vi "Format Page.vi"() -> ()   [LabVIEW 2020, in "2D Plot.lvclass"]
uses:
  <vilib>/Math Plots/2D Math Plots/2D Plot/2D Plot/2D Plot.lvclass
  <vilib>/Math Plots/2D Math Plots/2D Plot/Action String/2DMathPlot Ctrl Act Queue.ctl
  <vilib>/Math Plots/2D Math Plots/2D Plot/Action String/2DMathPlot Ctrl Act Cluster.ctl
  <vilib>/Math Plots/2D Math Plots/2D Plot/Action String/2DMathPlot State Class.ctl
  <vilib>/Math Plots/2D Math Plots/2D Plot/2D Plot/Typedef/Dialog State.ctl
  <vilib>/Math Plots/2D Math Plots/2D Plot/2D Plot/Typedef/Temp Graph State.ctl
  <vilib>/Math Plots/2D Math Plots/2D Plot/2D Plot/Typedef/Temp Graph Property Action.ctl
panel:
  in  "R Axis":string="(R-Axis)"
  in  "Axis":string[](array[string])=["(X-Axis)", "(Y-Axis)"]
  in  "Control Ref Queue":T1
  out "Format String Out":string[](array[string])
  in  "Format String In":string[](array[string])
  out "Format test string":string
  in  "Caption Texts":string[](array[string])=["Numeric Format Codes", "Absolute Time Format Codes\n(must be within %< >T)", "Relative Time Format Codes\n(must be within %< >t)"]
  in  "Item Names":string[][][](array[string])=[[["Floating point notation", "%f"], ["Scientific notation", "%e"], ["Engineering notation", "%^e"], ["Automatic notation", "%#_g"], ["SI notation", "%p"], ["Decimal", "%d"], ["Unsigned decimal", "%u"], ["Hexadecimal", "%x"], ["Octal", "%o"], ["Binary", "%b"], ["A single percent character", "%%"], ["", ""], ["", ""], ["", ""], ["", ""], ["", ""], ["", ""], ["", ""], ["", ""], ["", ""], ["", ""], ["", ""], ["", ""]], [["Absolute time container", "%< >T"], ["Abbreviated weekday name", "%a"], ["Weekday name", "%A"], ["Abbreviated month name", "%b"], ["Month name", "%B"], ["Default date and time", "%c"], ["Day of month (01-31)", "%d"], ["Hour (24-hour clock) (00-23)", "%H"], ["Hour (12-hour clock) (01-12)", "%I"], ["Day of year (001-366)", "%j"], ["Month number (01-12)", "%m"], ["Minute (00-59)", "%M"], ["AM or PM flag", "%p"], ["Seconds (00-59)", "%S"], ["Fractional seconds with <digit>\nprecision", "%<digit> u"], ["Week number (00-53) with\nSunday as the first day of week 1", "%U"], ["Weekday number (0-6)", "%w"], ["Week number (00-53) with\nMonday as the first day of week 1", "%W"], ["Locale date", "%x"], ["Locale time", "%X"], ["Year within century (00-99)", "%y"], ["Year including century", "%Y"], ["Time zone", "%Z"]], [["Relative time container", "%< >t"], ["Weeks", "%W"], ["Days", "%D"], ["Hours", "%H"], ["Minutes", "%M"], ["Seconds", "%S"], ["Fractional seconds with <digit>\nprecision", "%<digit>u"], ["A single percent character", "%%"], ["", ""], ["", ""], ["", ""], ["", ""], ["", ""], ["", ""], ["", ""], ["", ""], ["", ""], ["", ""], ["", ""], ["", ""], ["", ""], ["", ""], ["", ""]]]
  out "Advanced Tab":enum32{"Standard", "Advanced"}(tab)
  out "Time/Date Tab":enum32{"numeric", "time"}(tab) caption="Tab Control 3"
  in  "HLP_just/pad":i32(ring) items=["Pad with spaces on left", "Pad with spaces on right", "Pad with zeros on left"]
  in  "HLP_UseMinWidth":bool caption="Use minimum field width"
  in  "HLP_trailing zeros":bool caption="Hide trailing zeros"
  in  "HLP_exponent":bool caption="Exponent in multiples of 3"
  in  "Precision Type":u16(ring) items=["Digits of precision", "Significant digits"]
  in  "Digits":i32 min=0
  in  "HLP_Minimum field width":i32 caption="Minimum field width" min=0
  in  "HLP_year-new":T2(radio)
  in  "HLP_MDY 2-new":T2(radio)
  in  "HLP_HMS-new":enum32{"Radio Selection 1", "Radio Selection 2"}(radio)
  in  "HLP_Hour Type-new":enum32{"Radio Selection 1", "Radio Selection 2"}(radio)
  in  "HLP_Date Type":u16(ring)=1 caption="Date Type" items=["Custom date format", "System date format", "Date unused"]
  in  "HLP_Digits":i32 caption="Digits" min=0
  in  "HLP_Time Type":u16(ring)=1 caption="Time Type" items=["Custom time format", "System time format", "Time unused"]
  in  "Type":i32(listbox)
  in  "HLP_Revert":bool caption="Revert"
  in  "HLP_Format Code List Type":u16(ring) items=["Numeric format codes", "Relative time format codes", "Absolute time format codes"]
  out "HLP_Valid Fmt String":bool=TRUE caption="Valid"
  in  "HLP_insert format code":bool caption="Insert into Format String"
  in  "HLP_percent codes":i32(listbox) caption="Numeric Format Codes"
  in  "ODF_Format String":string caption="Format string"
  in  "HLP_AdvancedFmt2":enum32{"Default mode", "Advanced mode"}(radio)
  in  "Current Scale":u16(ring) items=["Time", "Amplitude"]
  in  "Event Registration":refnum<event-registration>
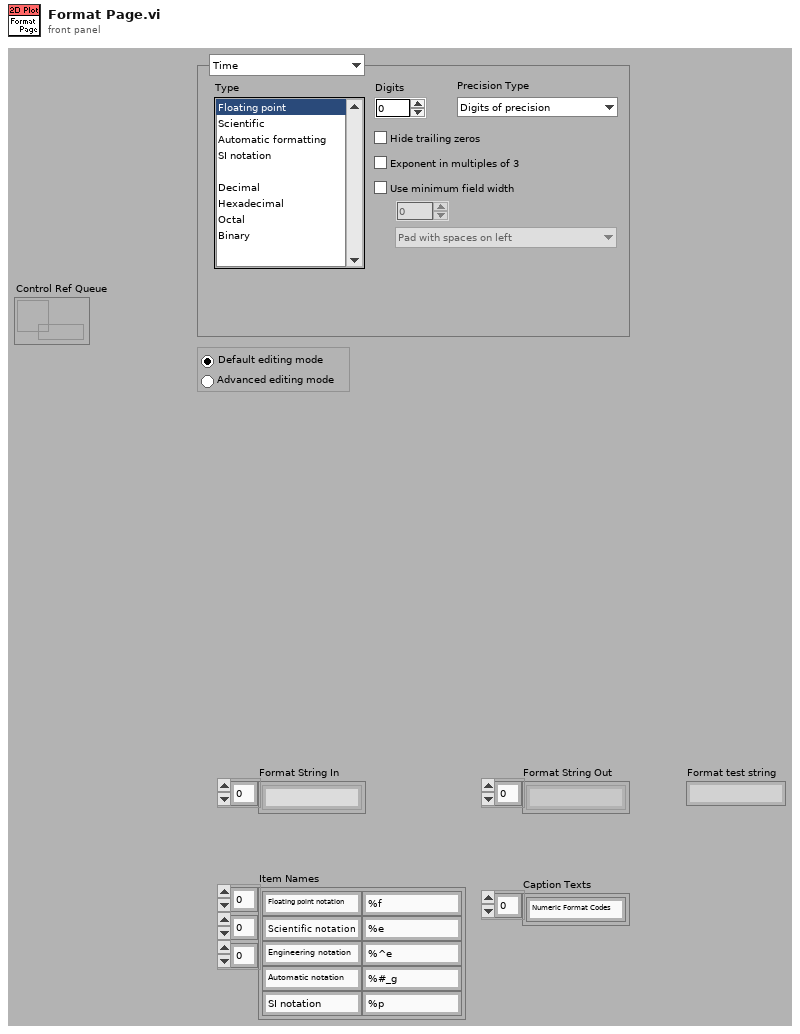
[diagram p1: front panel]
types:
  T1 = typedef "2DMathPlot Ctrl Act Queue.ctl" = refnum<queue>
  T2 = enum32{"Radio Selection 1", "Radio Selection 2", "Radio Selection 3"}
  T3 = typedef "2D Plot.lvclass/Dialog State.ctl" = enum16{"Initialize", "Read Property", "Write Property", "Idle", "Exit"}
  T4 = typedef "2D Plot.lvclass/Temp Graph State.ctl" = enum16{"Create", "Update Graph", "Update Property Only", "Get Plot Name", "Get Axis Name", "Destory"}
  T5 = typedef "2D Plot.lvclass/Temp Graph Property Action.ctl" = enum16{"Appearance Property", "Format Property", "Plots Property", "Scales Property"}
  T6 = enum16{"number", "absolute time", "relative time"}
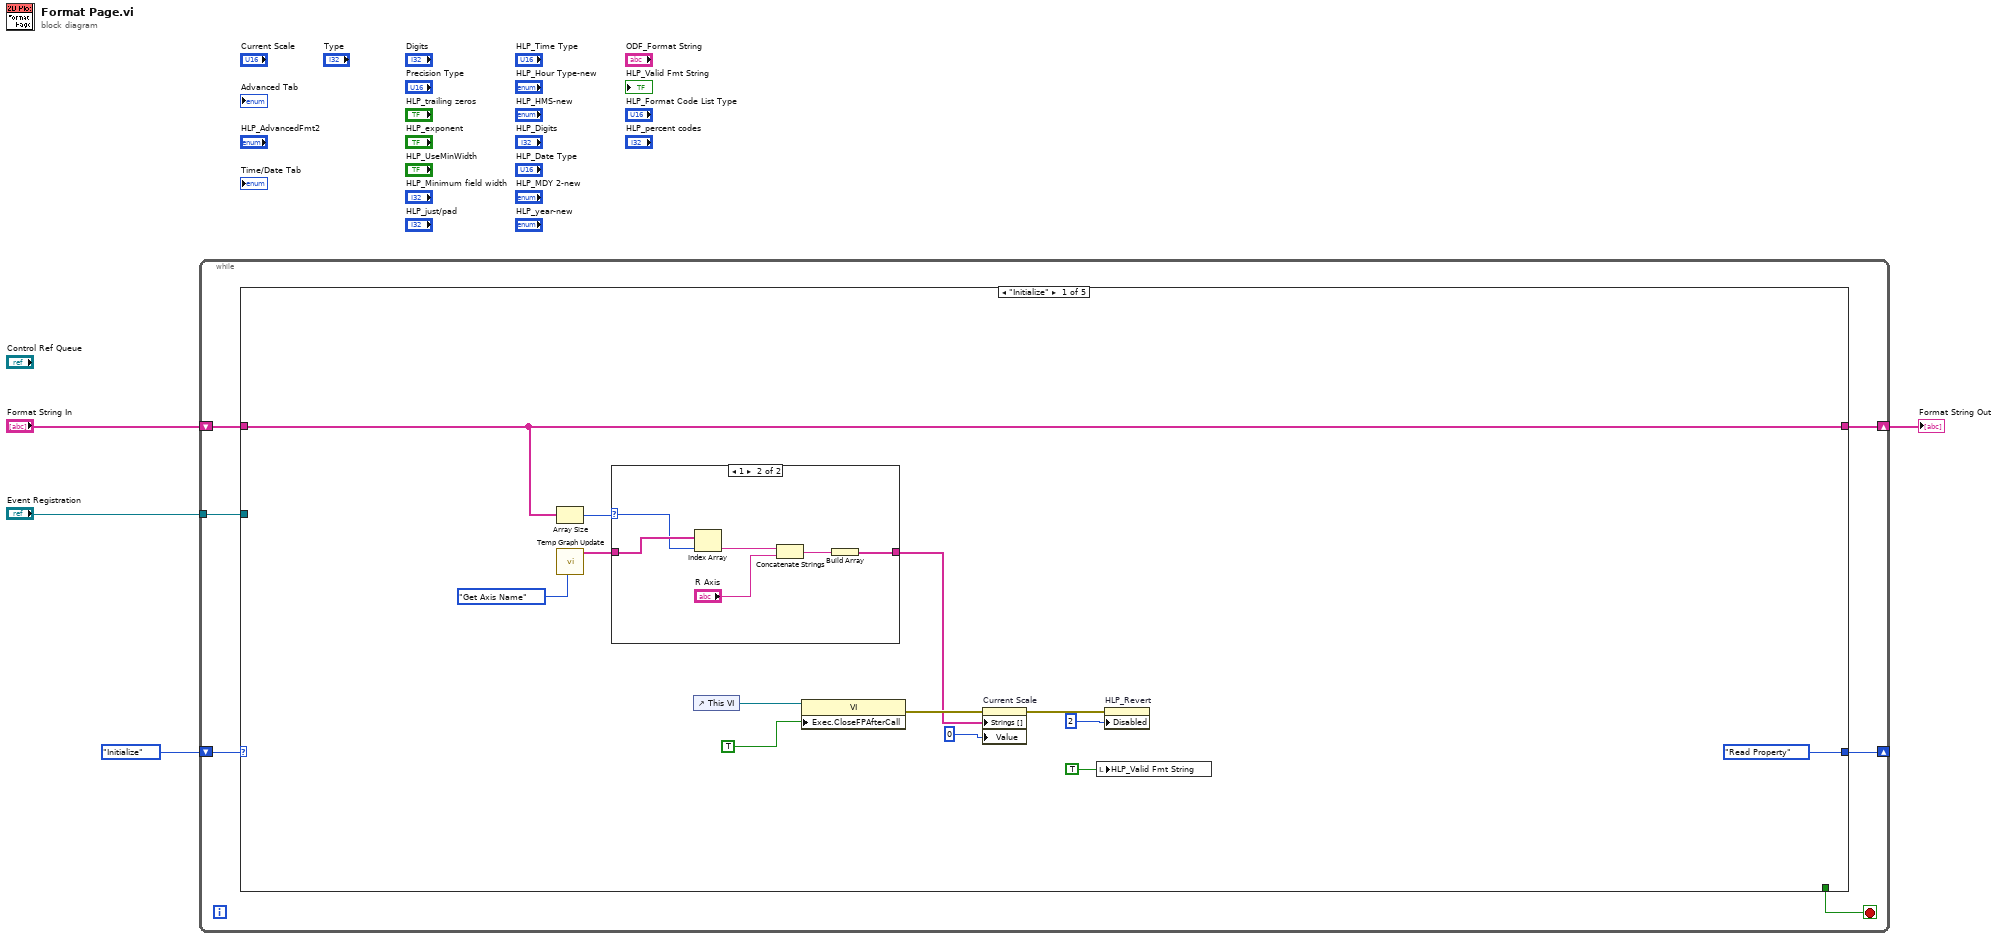
[diagram p0: block diagram]
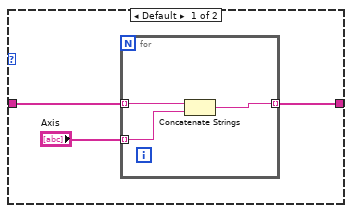
[diagram p2: hidden frame]
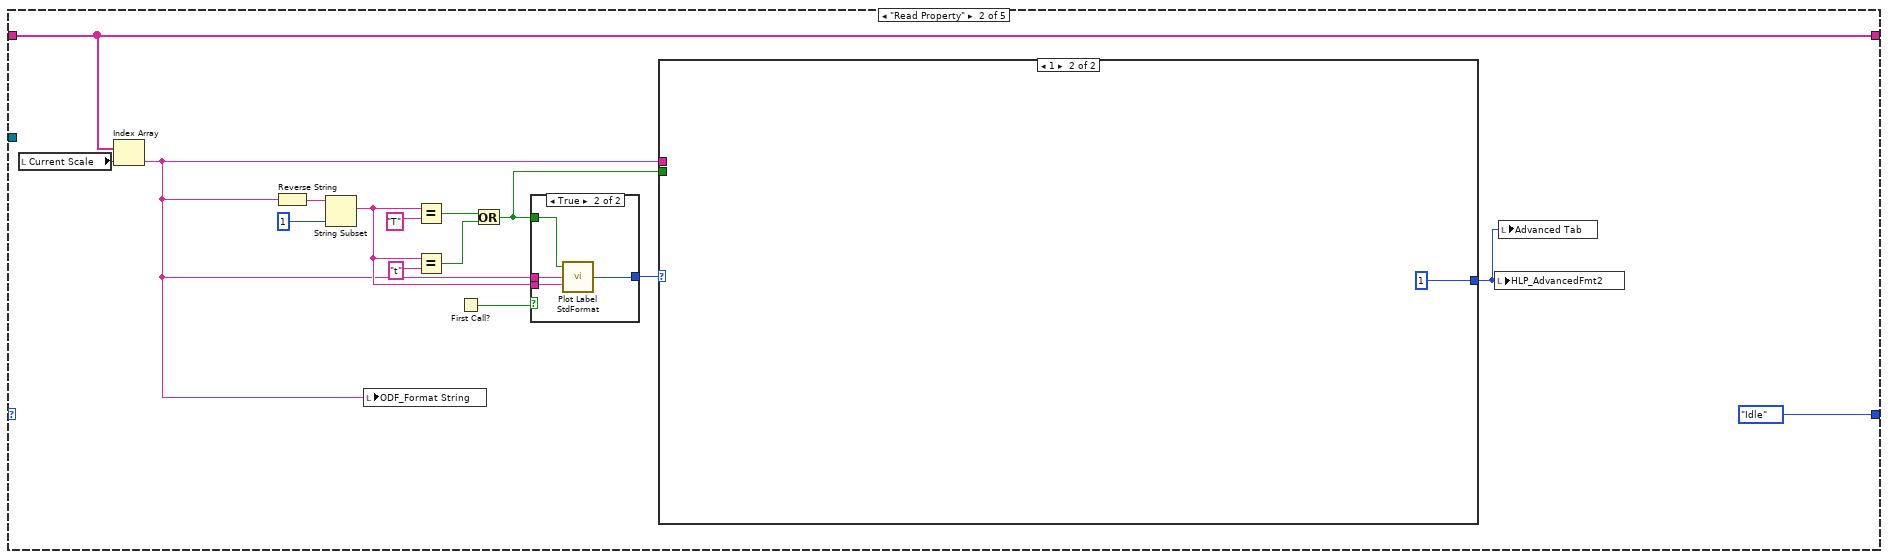
[diagram p3: hidden frame]
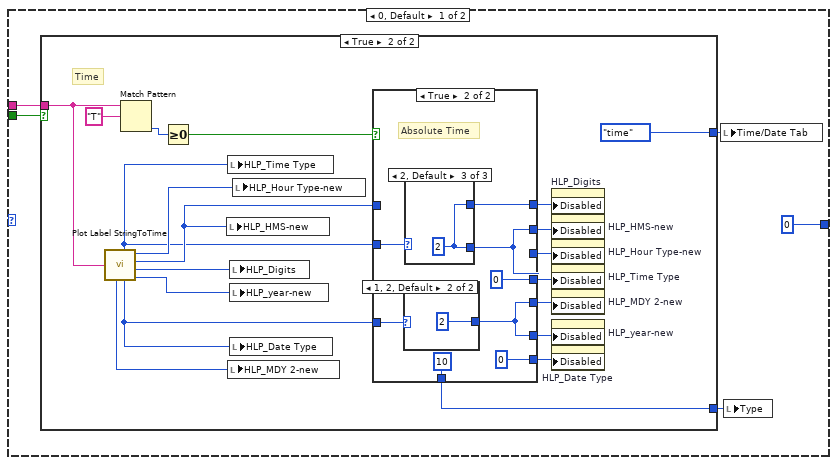
[diagram p4: hidden frame]
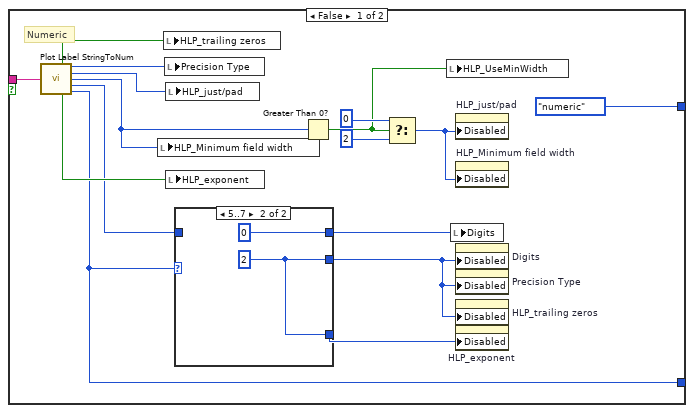
[diagram p5: hidden frame]
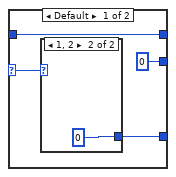
[diagram p6: hidden frame]
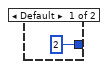
[diagram p7: hidden frame]
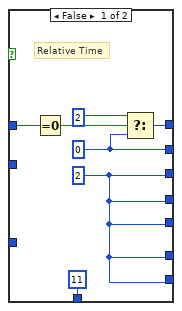
[diagram p8: hidden frame]
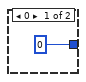
[diagram p9: hidden frame]
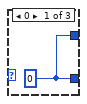
[diagram p10: hidden frame]
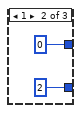
[diagram p11: hidden frame]
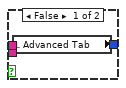
[diagram p12: hidden frame]
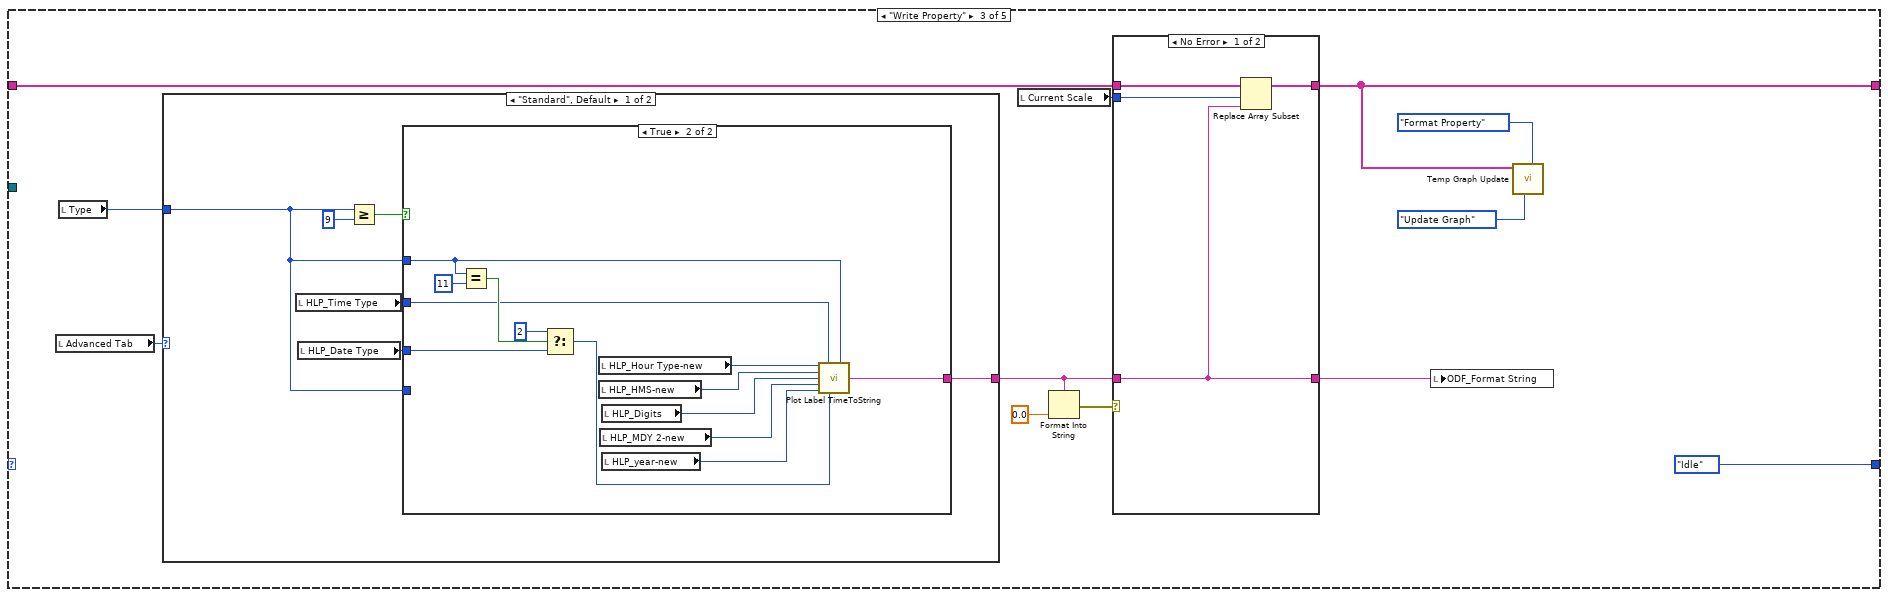
[diagram p13: hidden frame]
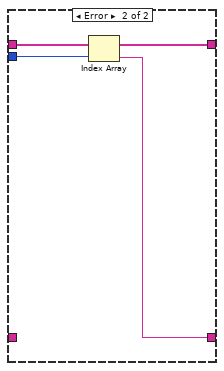
[diagram p14: hidden frame]
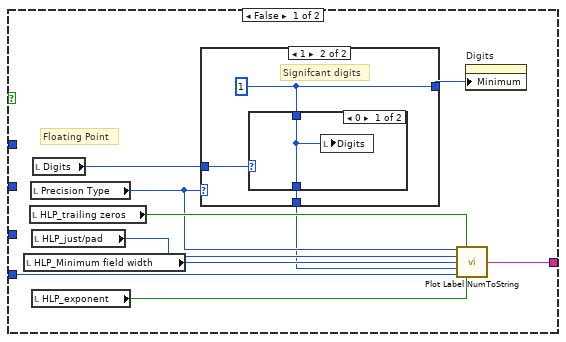
[diagram p15: hidden frame]
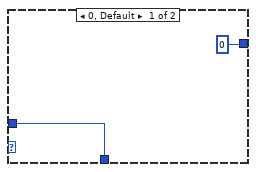
[diagram p16: hidden frame]
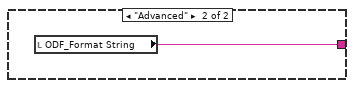
[diagram p18: hidden frame]
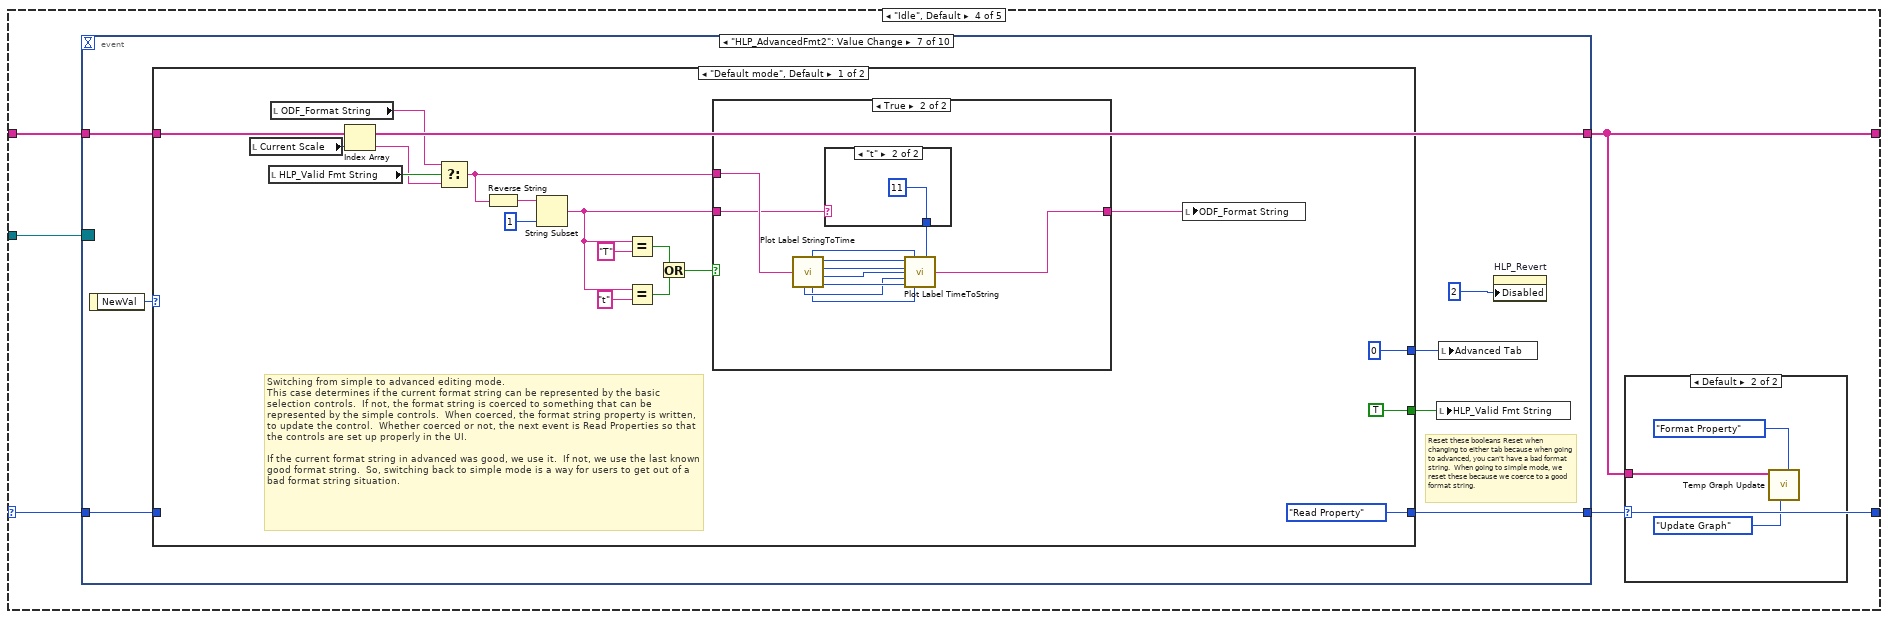
[diagram p19: hidden frame]
diagram:
  n1 = while {
    shift-right: [w5] -> w2
    shift-left: "Format String In" -> [w10]
    shift-right: [w6] -> _
    shift-left: Dialog_State."Initialize" ("Enum") -> [w7]
    tunnel: "Event Registration" -> [w8]
    stop <- w9 stop-if-true
    n2 = case shown="\"Initialize\"" w7 {
      selector: w7 -> [_ _ _ w185 _]
      tunnel: w10 -> [w15 w49 w130 w187 w410]
      tunnel: [w15 w49 w127 w184 w410] -> w5
      tunnel: [Dialog_State."Read Property" ("Enum") Dialog_State."Idle" ("Enum") Dialog_State."Idle" ("Enum") w183 Dialog_State."Exit" ("Enum")] -> w6
      tunnel: [_ _ _ _ TRUE] -> w9
      tunnel: w8 -> [_ _ _ w186 _]
      frame "Initialize" {
        n3 = Array Size(array=w15) -> (size(s)=w12:i32)
        n4 = call <vilib>:"Temp Graph Update.vi"("State"=Temp_Graph_State."Get Axis Name") -> ("Item Strings"=w14:string[])  [unwired: 4 in, 6 out]
        n5 = case shown="1" w12 {
          selector: w12 -> [_ w34]
          tunnel: w14 -> [w26 w35]
          tunnel: [w24 w30] -> w13
          frame Default {
            n6 = for {
              tunnel: w26 -> [w29] mode=indexing
              tunnel: "Axis" -> [w28] mode=indexing
              tunnel: [w27] -> w24 mode=indexing
              n7 = Concatenate Strings(w29, w28) -> (w27:string)
            }
          }
          frame 1 {
            n8 = Index Array(array=w35, index=w34) -> (element=w33:string)
            n9 = Concatenate Strings(w33, "R Axis") -> (w31:string)
            n10 = Build Array(w31) -> (w30:string[])
          }
        }
        n11 = control-ref of="This VI"() -> (w23:refnum<vi>)
        n12 = property class="VI"(reference=w23, "Exec.CloseFPAfterCall"=TRUE ("Execution:Close After Call")) -> (error out=w18:errorcluster)  [unwired: 1 in, 1 out]
        n13 = property on="Current Scale" class="Ring (strict)"(error in=w18, "Strings []"=w13, "Value"=u16 0) -> (error out=w17:errorcluster)  [unwired: 1 in, 1 out]
        n14 = local write "HLP_Valid Fmt String"(TRUE ("HLP_Valid Fmt String")) -> ()
        n15 = property on="HLP_Revert" class="Bool"(error in=w17, "Disabled"=u8 2) -> ()  [unwired: 1 in, 2 out]
      }
      frame "Read Property" {
        n16 = local read "Current Scale"() -> (w50:u16)
        n17 = Index Array(array=w49, index=w50) -> (element=w39:string)
        n18 = Reverse String(1:w39) -> (0:w44:string)
        n19 = String Subset(string=w44, length (rest)=1 ("length (rest)")) -> (substring=w48:string)  [unwired: 1 out]
        n20 = local write "ODF_Format String"(w39) -> ()
        n21 = Equal?(x=w48, y="T") -> (x = y?=w46:bool)
        n22 = Equal?(x=w48, y="t") -> (x = y?=w47:bool)
        n23 = First Call?() -> (First Call?: T/F=w41:bool)
        n24 = Or(x=w46, y=w47) -> (x .or. y?=w38:bool)
        n25 = case shown="True" w41 {
          tunnel: w48 -> [_ w124]
          tunnel: w38 -> [_ w126]
          tunnel: w39 -> [_ w125]
          tunnel: [w122 w123] -> w40
          frame False {
            n26 = local read "Advanced Tab"() -> (w122:enum32{"Standard", "Advanced"})
          }
          frame True {
            n27 = call <vilib>:"Plot Label StdFormat.vi"("Time Type"=w124, "Format String"=w125, "Type (false = numeric)"=w126) -> ("Custom"=w123:i32)
          }
        }
        n28 = case shown="1" w40 {
          tunnel: w39 -> [w55 _]
          tunnel: w38 -> [w54 _]
          tunnel: [0 1] -> w37
          frame 0, Default {
            n29 = case shown="True" w54 {
              tunnel: w55 -> [w71 w97]
              tunnel: [w64 w88] -> w53
              tunnel: [enum32{"numeric", "time"}."numeric" ("Time/Date Tab") enum32{"numeric", "time"}."time" ("Time/Date Tab")] -> w52
              frame False {
                # "Numeric"
                n30 = call <vilib>:"Plot Label StringToNum.vi"("Format String"=w71) -> ("Hide trailing zeros"=w70:bool, "Digit Type"=w68:i32, "just/pad"=w67:i32, "Minimum Field Width"=w59:i32, "Digits of Precision"=w66:i32, "exponent"=w69:bool, "Numeric Format"=w64:i32)  [unwired: 8 out]
                n31 = local write "HLP_Minimum field width"(w59) -> ()
                n32 = local write "HLP_trailing zeros"(w70) -> ()
                n33 = local write "Precision Type"(w68) -> ()
                n34 = local write "HLP_just/pad"(w67) -> ()
                n35 = local write "HLP_exponent"(w69) -> ()
                n36 = case shown="5..7" w64 {
                  selector: w64 -> [w73 _]
                  tunnel: [u8 0 w78] -> w63
                  tunnel: w66 -> [w74 _]
                  tunnel: [w74 0 ("Digits of Precision")] -> w65
                  tunnel: [w72 w78] -> w62
                  frame Default {
                    n37 = case shown="1, 2" w73 {
                      tunnel: [u8 2 u8 0] -> w72
                      frame Default {
                      }
                      frame 1, 2 {
                      }
                    }
                  }
                  frame 5..7 {
                    w78 = u8 2
                  }
                }
                n38 = Greater Than 0?(x=w59) -> (x > 0?=w58:bool)
                n39 = Select(t=u8 0, s=w58, f=u8 2) -> (s? t:f=w57:u8)
                n40 = local write "HLP_UseMinWidth"(w58) -> ()
                n41 = local write "Digits"(w65) -> ()
                n42 = property on="HLP_just/pad" class="Ring (strict)"("Disabled"=w57) -> ()  [unwired: 2 in, 2 out]
                n43 = property on="HLP_Minimum field width" class="DigNum (strict)"("Disabled"=w57) -> ()  [unwired: 2 in, 2 out]
                n44 = property on="Digits" class="DigNum (strict)"("Disabled"=w63) -> ()  [unwired: 2 in, 2 out]
                n45 = property on="Precision Type" class="Ring (strict)"("Disabled"=w63) -> ()  [unwired: 2 in, 2 out]
                n46 = property on="HLP_trailing zeros" class="Bool (strict)"("Disabled"=w63) -> ()  [unwired: 2 in, 2 out]
                n47 = property on="HLP_exponent" class="Bool (strict)"("Disabled"=w62) -> ()  [unwired: 2 in, 2 out]
              }
              frame True {
                # "Time"
                n48 = call <vilib>:"Plot Label StringToTime.vi"("Time & Date Format String"=w97) -> ("MDY"=w95:i16, "Time Format"=w91:i16, "AM/PM"=w96:i16, "included seconds"=w92:i16, "Date Format"=w90:i16, "seconds precision"=w93:i16, "Year Format"=w94:i16)  [unwired: 3 out]
                n49 = Match Pattern(string=w97, regular expression="T") -> (offset past match=w99:i32)  [unwired: 4 out]
                n50 = Greater Or Equal To 0?(x=w99) -> (x >= 0?=w89:bool)
                n51 = local write "HLP_HMS-new"(w92) -> ()
                n52 = local write "HLP_Time Type"(w91) -> ()
                n53 = local write "HLP_MDY 2-new"(w95) -> ()
                n54 = local write "HLP_Digits"(w93) -> ()
                n55 = local write "HLP_year-new"(w94) -> ()
                n56 = local write "HLP_Date Type"(w90) -> ()
                n57 = local write "HLP_Hour Type-new"(w96) -> ()
                n58 = case shown="True" w89 {
                  tunnel: [w101 w114] -> w85
                  tunnel: [w106 w114] -> w84
                  tunnel: [w100 w107] -> w86
                  tunnel: [w106 0] -> w83
                  tunnel: [w106 0] -> w80
                  tunnel: [w106 w111] -> w81
                  tunnel: [w106 w111] -> w82
                  tunnel: w91 -> [_ w110]
                  tunnel: w90 -> [_ w109]
                  tunnel: [11 10] -> w88
                  tunnel: w92 -> [w102 _]
                  frame False {
                    w101 = 0
                    w106 = 2
                    # "Relative Time"
                    n59 = Equal To 0?(x=w102) -> (x = 0?=w103:bool)
                    n60 = Select(t=2, s=w103, f=w101) -> (s? t:f=w100:i32)
                  }
                  frame True {
                    # "Absolute Time"
                    n61 = case shown="1, 2, Default" w109 {
                      tunnel: [0 2] -> w111
                      frame 0 {
                      }
                      frame 1, 2, Default {
                      }
                    }
                    n62 = case shown="2, Default" w110 {
                      tunnel: [w117 2 w120] -> w114
                      tunnel: [w117 0 w120] -> w107
                      frame 0 {
                        w117 = 0
                      }
                      frame 1 {
                      }
                      frame 2, Default {
                        w120 = 2
                      }
                    }
                  }
                }
                n63 = property on="HLP_Digits" class="DigNum (strict)"("Disabled"=w86) -> ()  [unwired: 2 in, 2 out]
                n64 = property on="HLP_HMS-new" class="RadioBtnsControl (strict)"("Disabled"=w85) -> ()  [unwired: 2 in, 2 out]
                n65 = property on="HLP_Hour Type-new" class="RadioBtnsControl (strict)"("Disabled"=w84) -> ()  [unwired: 2 in, 2 out]
                n66 = property on="HLP_Time Type" class="Ring (strict)"("Disabled"=w83) -> ()  [unwired: 2 in, 2 out]
                n67 = property on="HLP_MDY 2-new" class="RadioBtnsControl (strict)"("Disabled"=w82) -> ()  [unwired: 2 in, 2 out]
                n68 = property on="HLP_year-new" class="RadioBtnsControl (strict)"("Disabled"=w81) -> ()  [unwired: 2 in, 2 out]
                n69 = property on="HLP_Date Type" class="Ring (strict)"("Disabled"=w80) -> ()  [unwired: 2 in, 2 out]
              }
            }
            n70 = local write "Time/Date Tab"(w52) -> ()
            n71 = local write "Type"(w53) -> ()
          }
          frame 1 {
          }
        }
        n72 = local write "HLP_AdvancedFmt2"(w37) -> ()
        n73 = local write "Advanced Tab"(w37) -> ()
      }
      frame "Write Property" {
        n74 = local read "Advanced Tab"() -> (w138:enum32{"Standard", "Advanced"})
        n75 = local read "Type"() -> (w137:i32)
        n76 = case shown="\"Standard\", Default" w138 {
          tunnel: w137 -> [w149 _]
          tunnel: [w146 w182] -> w134
          frame "Standard", Default {
            n77 = local read "HLP_Time Type"() -> (w148:u16)
            n78 = local read "HLP_Date Type"() -> (w147:u16)
            n79 = Greater Or Equal?(x=w149, y=9) -> (x >= y?=w150:bool)
            n80 = case shown="True" w150 {
              tunnel: w149 -> [_ w176]
              tunnel: w149 -> [w160 _]
              tunnel: w148 -> [_ w177]
              tunnel: w147 -> [_ w178]
              tunnel: [w161 w169] -> w146
              frame False {
                # "Floating Point"
                n81 = local read "HLP_Minimum field width"() -> (w158:i32)
                n82 = local read "HLP_trailing zeros"() -> (w157:bool)
                n83 = local read "Precision Type"() -> (w155:u16)
                n84 = local read "HLP_just/pad"() -> (w156:i32)
                n85 = local read "HLP_exponent"() -> (w159:bool)
                n86 = local read "Digits"() -> (w154:i32)
                n87 = case shown="1" w155 {
                  tunnel: w154 -> [w162 w166]
                  tunnel: [0 ("Data Range:Minimum") w165] -> w153
                  tunnel: [w162 w164] -> w152
                  frame 0, Default {
                  }
                  frame 1 {
                    w165 = 1 ("Data Range:Minimum")
                    # "Signifcant digits"
                    n88 = case shown="0" w166 {
                      selector: w166 -> [_ w168]
                      tunnel: w165 -> [w167 _]
                      tunnel: [w167 w168] -> w164
                      frame 0 {
                        n89 = local write "Digits"(w167) -> ()
                      }
                      frame 1, Default {
                      }
                    }
                  }
                }
                n90 = call <vilib>:"Plot Label NumToString.vi"("Digit Type"=w155, "Hide trailing zeros"=w157, "just/pad"=w156, "Minimum Field Width"=w158, "Digits of Precision"=w152, "Numeric Format"=w160, "exponent"=w159) -> ("Format String"=w161:string)  [unwired: 8 out]
                n91 = property on="Digits" class="DigNum (strict)"("Minimum"=w153) -> ()  [unwired: 2 in, 2 out]
              }
              frame True {
                n92 = Equal?(x=w176, y=11) -> (x = y?=w179:bool)
                n93 = Select(t=u16 2, s=w179, f=w178) -> (s? t:f=w170:u16)
                n94 = local read "HLP_Hour Type-new"() -> (w175:enum32{"Radio Selection 1", "Radio Selection 2"})
                n95 = local read "HLP_HMS-new"() -> (w174:enum32{"Radio Selection 1", "Radio Selection 2"})
                n96 = local read "HLP_MDY 2-new"() -> (w172:T2)
                n97 = local read "HLP_Digits"() -> (w173:i32)
                n98 = local read "HLP_year-new"() -> (w171:T2)
                n99 = call <vilib>:"Plot Label TimeToString.vi"("AM/PM"=w175, "Time Format"=w177, "Type (10 = Absolute)"=w176, "included seconds"=w174, "seconds precision"=w173, "m-d-y sequence"=w172, "year format"=w171, "Date Format"=w170) -> ("Format String"=w169:string)  [unwired: 3 in, 4 out]
              }
            }
          }
          frame "Advanced" {
            n100 = local read "ODF_Format String"() -> (w182:string)
          }
        }
        n101 = local read "Current Scale"() -> (w133:u16)
        n102 = Format Into String(format string=w134, 0.0 ("input 1")) -> (error out=w135:errorcluster)  [unwired: 2 in, 1 out]
        n103 = case shown="No Error" w135 {
          tunnel: w130 -> [w142 w143]
          tunnel: [w141 w143] -> w127
          tunnel: w134 -> [w139 _]
          tunnel: w133 -> [w140 w145]
          tunnel: [w139 w144] -> w132
          frame No Error {
            n104 = Replace Array Subset(array=w142, new element=w139, index=w140) -> (w141:string[])
          }
          frame Error {
            n105 = Index Array(array=w143, index=w145) -> (element=w144:string)
          }
        }
        n106 = local write "ODF_Format String"(w132) -> ()
        n107 = call <vilib>:"Temp Graph Update.vi"("Property Name"=Temp_Graph_Property_Action."Format Property", "State"=Temp_Graph_State."Update Graph", "Property In"=w127) -> ()  [unwired: 2 in, 7 out]
      }
      frame "Idle", Default {
        n108 = event shown="[6] \"HLP_AdvancedFmt2\": Value Change" {
          selector: w186 -> [_ _ _ _ _ _ _ _ _ _]
          dyn-events: _ -> [_ _ _ _ _ _ _ _ _ _]
          timeout: _ -> [_ _ _ _ _ _ _ _ _ _]
          tunnel: w187 -> [w192 w194 w198 w269 w297 w303 w313 w381 w388 w408]
          tunnel: [w192 w194 w198 w268 w297 w303 w313 w381 w388 w408] -> w184
          tunnel: [Dialog_State."Read Property" ("Enum") Dialog_State."Write Property" ("Enum") Dialog_State."Write Property" ("Enum") w276 w298 Dialog_State."Write Property" ("Enum") w309 w380 w387 Dialog_State."Exit" ("Enum")] -> w183
          tunnel: w185 -> [_ _ _ w276 w298 _ w308 w380 w387 _]
          event "Current Scale": Value Change {
            n109 = event-data() -> ()  [unwired: 7 out]
          }
          event "HLP_Digits", "Digits", "HLP_just/pad", "HLP_exponent", "HLP_trailing zeros", "Precision Type", "HLP_Hour Type-new", "HLP_MDY 2-new", "HLP_year-new": Value Change {
            n110 = event-data() -> ()  [unwired: 7 out]
          }
          event "HLP_Date Type", "HLP_Time Type", "Type", "HLP_Minimum field width", "HLP_HMS-new": Value Change {
            n111 = event-data() -> ()  [unwired: 7 out]
            n112 = local read "HLP_AdvancedFmt2"() -> (w200:enum32{"Default mode", "Advanced mode"})
            n113 = local read "Type"() -> (w196:i32)
            n114 = case shown="6..8" w196 {
              selector: w196 -> [w201 _]
              tunnel: [w201 u8 5] -> w195
              frame Default {
              }
              frame 6..8 {
              }
            }
            n115 = local write "Type"(w195) -> ()
            n116 = case shown="\"Default mode\", Default" w200 {
              tunnel: w195 -> [w210 _]
              tunnel: [u32 0 u32 1] -> w199
              frame "Default mode", Default {
                n117 = case shown="5..8" w210 {
                  selector: w210 -> [w259 _]
                  tunnel: [u8 0 w264] -> w219
                  tunnel: [w260 w264] -> w220
                  frame Default {
                    n118 = case shown="1, 2" w259 {
                      tunnel: [u8 2 u8 0] -> w260
                      frame Default {
                      }
                      frame 1, 2 {
                      }
                    }
                  }
                  frame 5..8 {
                    w264 = u8 2
                  }
                }
                n119 = Greater Or Equal?(x=w210, y=9) -> (x >= y?=w222:bool)
                n120 = Equal?(x=w210, y=11) -> (x = y?=w211:bool)
                n121 = Boolean To (0,1)(Boolean=w222) -> (0, 1=w221:i16)
                n122 = local write "Time/Date Tab"(w221) -> ()
                n123 = property on="HLP_exponent" class="Bool (strict)"("Disabled"=w220) -> ()  [unwired: 2 in, 2 out]
                n124 = property on="Precision Type" class="Ring (strict)"("Disabled"=w219) -> ()  [unwired: 2 in, 2 out]
                n125 = property on="HLP_trailing zeros" class="Bool (strict)"("Disabled"=w219) -> ()  [unwired: 2 in, 2 out]
                n126 = property on="Digits" class="DigNum (strict)"("Disabled"=w219) -> ()  [unwired: 2 in, 2 out]
                n127 = local read "HLP_Minimum field width"() -> (w216:i32)
                n128 = case shown="True" w211 {
                  tunnel: [w229 w255] -> w209
                  tunnel: [w228 w254] -> w208
                  tunnel: [w224 w253] -> w207
                  tunnel: [w227 w253] -> w206
                  tunnel: [w226 w253] -> w205
                  tunnel: [w225 w253] -> w204
                  tunnel: [w224 w253] -> w203
                  frame False {
                    w224 = u8 0
                    # "Absolute Time"
                    n129 = local read "HLP_Time Type"() -> (w231:u16)
                    n130 = local read "HLP_Date Type"() -> (w230:u16)
                    n131 = call <vilib>:"Plot subChangeDetector.vi"("value"=w231) -> ("changed?"=w232:bool)  [unwired: 10 out]
                    n132 = Equal?(x=2, y=w231) -> (x = y?=w235:bool)
                    n133 = Equal?(x=2, y=w230) -> (x = y?=w234:bool)
                    n134 = And(x=w235, y=w234) -> (x .and. y?=w233:bool)
                    n135 = case shown="True" w233 {
                      tunnel: w232 -> [_ w250]
                      tunnel: w231 -> [w242 _]
                      tunnel: w230 -> [w241 _]
                      tunnel: [w240 w249] -> w229
                      tunnel: [w239 w249] -> w228
                      tunnel: [w239 w249] -> w227
                      tunnel: [w238 w249] -> w226
                      tunnel: [w238 w249] -> w225
                      frame False {
                        n136 = case shown="2, Default" w242 {
                          tunnel: [w245 u8 2 w248] -> w239
                          tunnel: [w245 u8 0 w248] -> w240
                          frame 0 {
                            w245 = u8 0
                          }
                          frame 1 {
                          }
                          frame 2, Default {
                            w248 = u8 2
                          }
                        }
                        n137 = case shown="1, 2, Default" w241 {
                          tunnel: [u8 0 u8 2] -> w238
                          frame 0 {
                          }
                          frame 1, 2, Default {
                          }
                        }
                      }
                      frame True {
                        w249 = u8 2
                        n138 = case shown="False" w250 {
                          frame False {
                            w251 = u16 1 items=["Custom Date Format", "System Date Format", "Date Unused"] ("Date Type")
                            n139 = local write "HLP_Date Type"(w251) -> ()
                          }
                          frame True {
                            w252 = u16 1 items=["Custom Time Format", "System Time Format", "Time Unused"] ("Time Type")
                            n140 = local write "HLP_Time Type"(w252) -> ()
                          }
                        }
                      }
                    }
                  }
                  frame True {
                    w253 = u8 2
                    w254 = u8 0
                    # "Relative Time"
                    n141 = local read "HLP_HMS-new"() -> (w256:enum32{"Radio Selection 1", "Radio Selection 2"})
                    n142 = Equal To 0?(x=w256) -> (x = 0?=w258:bool)
                    n143 = Select(t=u8 2, s=w258, f=w254) -> (s? t:f=w255:u8)
                  }
                }
                n144 = Greater Than 0?(x=w216) -> (x > 0?=w215:bool)
                n145 = Select(t=u8 0, s=w215, f=u8 2) -> (s? t:f=w214:u8)
                n146 = local write "HLP_UseMinWidth"(w215) -> ()
                n147 = property on="HLP_Minimum field width" class="DigNum (strict)"("Disabled"=w214) -> ()  [unwired: 2 in, 2 out]
                n148 = property on="HLP_just/pad" class="Ring (strict)"("Disabled"=w214) -> ()  [unwired: 2 in, 2 out]
                n149 = property on="HLP_Digits" class="DigNum (strict)"("Disabled"=w209) -> ()  [unwired: 2 in, 2 out]
                n150 = property on="HLP_HMS-new" class="RadioBtnsControl (strict)"("Disabled"=w208) -> ()  [unwired: 2 in, 2 out]
                n151 = property on="HLP_Hour Type-new" class="RadioBtnsControl (strict)"("Disabled"=w206) -> ()  [unwired: 2 in, 2 out]
                n152 = property on="HLP_Time Type" class="Ring (strict)"("Disabled"=w207) -> ()  [unwired: 2 in, 2 out]
                n153 = property on="HLP_MDY 2-new" class="RadioBtnsControl (strict)"("Disabled"=w205) -> ()  [unwired: 2 in, 2 out]
                n154 = property on="HLP_year-new" class="RadioBtnsControl (strict)"("Disabled"=w204) -> ()  [unwired: 2 in, 2 out]
                n155 = property on="HLP_Date Type" class="Ring (strict)"("Disabled"=w203) -> ()  [unwired: 2 in, 2 out]
              }
              frame "Advanced mode" {
              }
            }
            n156 = local write "Advanced Tab"(w199) -> ()
          }
          event "ODF_Format String": Value Change {
            n157 = event-data() -> ("NewVal"=w267:string)  [unwired: 1 out]
            n158 = Format Into String(format string=w267, 0.0 ("input 1")) -> (resulting string=→"Format test string":string, error out=w270:errorcluster)  [unwired: 2 in]
            n159 = local read "HLP_Valid Fmt String"() -> (w273:bool)
            n160 = Unbundle By Name(w270) -> ("status"=w272:bool)
            n161 = Not(x=w273) -> (.not. x?=w274:bool)
            n162 = And(x=w274, y=w272) -> (x .and. y?=w271:bool)
            n163 = case shown="False" w271 {
              tunnel: w270 -> [w282 _]
              tunnel: w269 -> [w279 w292]
              tunnel: [w278 w292] -> w268
              tunnel: w267 -> [w277 _]
              frame False {
                n164 = case shown="Error" w282 {
                  tunnel: [TRUE FALSE] -> w281
                  tunnel: [u8 2 u8 0] -> w280
                  tunnel: w279 -> [w286 w289]
                  tunnel: [w285 w289] -> w278
                  tunnel: w277 -> [w284 _]
                  frame No Error {
                    n165 = local read "Current Scale"() -> (w283:u16)
                    n166 = Replace Array Subset(array=w286, new element=w284, index=w283) -> (w285:string[])
                  }
                  frame Error {
                  }
                }
                n167 = local write "HLP_Valid Fmt String"(w281) -> ()
                n168 = property on="HLP_Revert" class="Bool"("Disabled"=w280) -> ()  [unwired: 2 in, 2 out]
              }
              frame True {
              }
            }
          }
          event "HLP_Revert": Value Change {
            n169 = event-data() -> ()  [unwired: 7 out]
            n170 = local read "Current Scale"() -> (w296:u16)
            n171 = Index Array(array=w297, index=w296) -> (element=w295:string)
            n172 = local write "HLP_Valid Fmt String"(TRUE ("HLP_Valid Fmt String")) -> ()
            n173 = local write "ODF_Format String"(w295) -> ()
            n174 = property on="HLP_Revert" class="Bool"("Disabled"=u8 2) -> ()  [unwired: 2 in, 2 out]
          }
          event "HLP_UseMinWidth": Value Change {
            n175 = event-data() -> ("NewVal"=w302:bool)  [unwired: 1 out]
            n176 = case shown="True" w302 {
              tunnel: [u8 2 u8 0] -> w301
              tunnel: [0 1] -> w300
              frame False {
              }
              frame True {
              }
            }
            n177 = local write "HLP_Minimum field width"(w300) -> ()
            n178 = property on="HLP_just/pad" class="Ring (strict)"("Disabled"=w301) -> ()  [unwired: 2 in, 2 out]
            n179 = property on="HLP_Minimum field width" class="DigNum (strict)"("Disabled"=w301) -> ()  [unwired: 2 in, 2 out]
          }
          event "HLP_AdvancedFmt2": Value Change {
            # "Reset these booleans Reset when changing to either tab because when going to advanced, you can't have a bad format string.  When going to simple mode, we reset these because we coerce to a good format string."
            n180 = event-data() -> ("NewVal"=w314:enum32{"Default mode", "Advanced mode"})  [unwired: 1 out]
            n181 = case shown="\"Default mode\", Default" w314 {
              tunnel: w313 -> [w332 _]
              tunnel: [0 1] -> w312
              tunnel: [TRUE ("HLP_Valid Fmt String") TRUE ("HLP_Valid Fmt String")] -> w310
              tunnel: [Dialog_State."Read Property" ("Enum") w368] -> w309
              tunnel: w308 -> [_ w368]
              frame "Default mode", Default {
                # "Switching from simple to advanced editing mode.\nThis case determines if the current format string can be represented by the basic selection controls.  If not, the format string is coerced to something that can be represented by the simple controls.  When coerced, the format string property is written, to update the control.  Whether coerced or not, the next event is Read Properties so that the controls are set up properly in the UI.\n\nIf the current format string in advanced was good, we use it.  If not, we use the last known good format string.  So, switching back to simple mode is a way for users to get out of a bad format string situation."
                n182 = local read "Current Scale"() -> (w331:u16)
                n183 = local read "HLP_Valid Fmt String"() -> (w330:bool)
                n184 = local read "ODF_Format String"() -> (w318:string)
                n185 = Index Array(array=w332, index=w331) -> (element=w329:string)
                n186 = Select(t=w318, s=w330, f=w329) -> (s? t:f=w321:string)
                n187 = Reverse String(1:w321) -> (0:w328:string)
                n188 = String Subset(string=w328, length (rest)=1 ("length (rest)")) -> (substring=w320:string)  [unwired: 1 out]
                n189 = Equal?(x=w320, y="T") -> (x = y?=w325:bool)
                n190 = Equal?(x=w320, y="t") -> (x = y?=w326:bool)
                n191 = Or(x=w325, y=w326) -> (x .or. y?=w322:bool)
                n192 = case shown="True" w322 {
                  tunnel: w321 -> [w333 w365]
                  tunnel: w320 -> [_ w364]
                  tunnel: [w334 w362] -> w319
                  frame False {
                    n193 = call <vilib>:"Plot Label StdFormat.vi"("Format String"=w333) -> ("Custom"=w335:i32)  [unwired: 2 in]
                    n194 = case shown="1" w335 {
                      tunnel: [w336 w337] -> w334
                      tunnel: w333 -> [w336 w345]
                      frame 0, Default {
                        # "Not a custom value.  Keep\nformat"
                      }
                      frame 1 {
                        # "Custom format.  Coerce.\nNote, ideally the page should not\ncoerce unless the user changes format\nin the default page."
                        n195 = call <vilib>:"Plot Label StringToNum.vi"("Format String"=w345) -> ("Hide trailing zeros"=w338:bool, "Digit Type"=w343:i32, "just/pad"=w342:i32, "Minimum Field Width"=w341:i32, "Digits of Precision"=w340:i32, "exponent"=w339:bool, "Numeric Format"=w344:i32)  [unwired: 8 out]
                        n196 = case shown="Default" w344 {
                          tunnel: w344 -> [_ w354]
                          tunnel: w343 -> [_ w353]
                          tunnel: w342 -> [_ w352]
                          tunnel: w341 -> [_ w351]
                          tunnel: w340 -> [_ w350]
                          tunnel: w339 -> [_ w349]
                          tunnel: w338 -> [_ w348]
                          tunnel: ["%.0f" w347] -> w337
                          frame -1 {
                          }
                          frame Default {
                            n197 = call <vilib>:"Plot Label NumToString.vi"("Digit Type"=w353, "Hide trailing zeros"=w348, "just/pad"=w352, "Minimum Field Width"=w351, "Digits of Precision"=w350, "Numeric Format"=w354, "exponent"=w349) -> ("Format String"=w347:string)  [unwired: 8 out]
                          }
                        }
                      }
                    }
                  }
                  frame True {
                    n198 = call <vilib>:"Plot Label StringToTime.vi"("Time & Date Format String"=w365) -> ("MDY"=w356:i16, "Time Format"=w361:i16, "AM/PM"=w360:i16, "included seconds"=w359:i16, "Date Format"=w355:i16, "seconds precision"=w358:i16, "Year Format"=w357:i16)  [unwired: 3 out]
                    n199 = case shown="\"t\"" w364 {
                      tunnel: [10 11] -> w363
                      frame "T", Default {
                      }
                      frame "t" {
                      }
                    }
                    n200 = call <vilib>:"Plot Label TimeToString.vi"("AM/PM"=w360, "Time Format"=w361, "Type (10 = Absolute)"=w363, "included seconds"=w359, "seconds precision"=w358, "m-d-y sequence"=w356, "year format"=w357, "Date Format"=w355) -> ("Format String"=w362:string)  [unwired: 3 in, 4 out]
                  }
                }
                n201 = local write "ODF_Format String"(w319) -> ()
              }
              frame "Advanced mode" {
                # "Switching from advanced to simple editing mode.\nThis case sets up the correct advanced format string table based on format type.  \n\nDon't go to read or write properties because the advanced tab shows the format string and it should be kept up-to-date by other events."
                n202 = local read "Type"() -> (w376:i32)
                n203 = case shown="9" w376 {
                  tunnel: [T6."number" ("Enum") T6."absolute time" ("Enum") T6."relative time" ("Enum")] -> w375
                  frame 0, Default {
                  }
                  frame 9 {
                  }
                  frame 10 {
                  }
                }
                n204 = Index Array(array="Item Names", index (dim 0)=w375) -> (element=w371:string[][])  [unwired: 2 in]
                n205 = Index Array(array="Caption Texts", index=w375) -> (element=w372:string)
                n206 = property on="HLP_percent codes" class="MCListbox (strict)"("ItemNames"=w371, "Caption.Text"=w372) -> ()  [unwired: 2 in, 2 out]
              }
            }
            n207 = local write "HLP_Valid Fmt String"(w310) -> ()
            n208 = local write "Advanced Tab"(w312) -> ()
            n209 = property on="HLP_Revert" class="Bool"("Disabled"=u8 2) -> ()  [unwired: 2 in, 2 out]
          }
          event "HLP_Format Code List Type": Value Change {
            n210 = event-data() -> ("NewVal"=w382:u16)  [unwired: 1 out]
            n211 = local read "Item Names"() -> (w384:string[][][])
            n212 = local read "Caption Texts"() -> (w383:string[])
            n213 = Index Array(array=w384, index (dim 0)=w382) -> (element=w385:string[][])  [unwired: 2 in]
            n214 = Index Array(array=w383, index=w382) -> (element=w386:string)
            n215 = property on="HLP_percent codes" class="MCListbox (strict)"("ItemNames"=w385, "Caption.Text"=w386) -> ()  [unwired: 2 in, 2 out]
          }
          event "HLP_insert format code": Value Change; "HLP_percent codes": Double Click {
            n216 = event-data() -> ()  [unwired: 5 out]
            n217 = property on="HLP_percent codes" class="MCListbox (strict)"() -> (error out=w389:errorcluster, "ItemNames"=w404:string[][], "Value"=w402:i32)  [unwired: 2 in, 1 out]
            n218 = local read "ODF_Format String"() -> (w396:string)
            n219 = property on="ODF_Format String" class="Str"(error in=w389) -> (error out=w391:errorcluster, "Text.Selection Start"=w394:u32)  [unwired: 1 in, 1 out]
            n220 = Index Array(array=w404, index (row)=w402, index (col)=1 ("disabled index (col)")) -> (element=w393:string)
            n221 = String Length(string=w393) -> (length=w401:i32)
            n222 = Add(x=w401, y=w394) -> (x+y=w400:u32)
            n223 = Search/Split String(string=w396, offset (0)=w394) -> (substring before match=w398:string, match + rest of string=w397:string)  [unwired: 2 out]
            n224 = property on="ODF_Format String" class="Str"(error in=w391, "Text.Selection Start"=w400, "Text.Selection End"=w400, "Key Focus"=TRUE) -> (error out=w390:errorcluster)  [unwired: 1 in, 1 out]
            n225 = Concatenate Strings(w398, w393, w397) -> (w395:string)
            n226 = case shown="\"No Error\", Default" w395 {
              selector: w395 -> [_ w406]
              tunnel: w396 -> [w405 _]
              tunnel: [w405 w406] -> w392
              frame "Error" {
              }
              frame "No Error", Default {
              }
            }
            n227 = property on="ODF_Format String" class="Str"(error in=w390, "Val(Sgnl)"=w392) -> ()  [unwired: 1 in, 2 out]
          }
          event User Event {
            n228 = event-data() -> ()  [unwired: 6 out]
          }
        }
        n229 = case shown="Default" w183 {
          tunnel: w184 -> [_ w189]
          frame "Write Property", "Exit" {
          }
          frame Default {
            n230 = call <vilib>:"Temp Graph Update.vi"("Property Name"=Temp_Graph_Property_Action."Format Property", "State"=Temp_Graph_State."Update Graph", "Property In"=w189) -> ()  [unwired: 2 in, 7 out]
          }
        }
      }
      frame "Exit" {
      }
    }
  }
  "Format String Out" <- w2
